vi "Comm String Send Command.vi"(0 "niDTS Comm String in":refnum<class "niDTS Comm String.lvclass">, 5 "Command":string, 7 "Args":string, 11 "error in (no error)":errorcluster) -> (4 "niDTS Comm String out":refnum<class "niDTS Comm String.lvclass">, 6 "Response":string, 15 "error out":errorcluster)   [LabVIEW 2015, in "niDTS CommLib.lvlib" / "niDTS Comm String.lvclass"]
uses:
  niDTS Comm String.lvclass
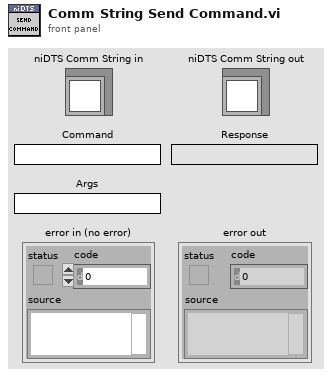
[diagram p1: front panel]
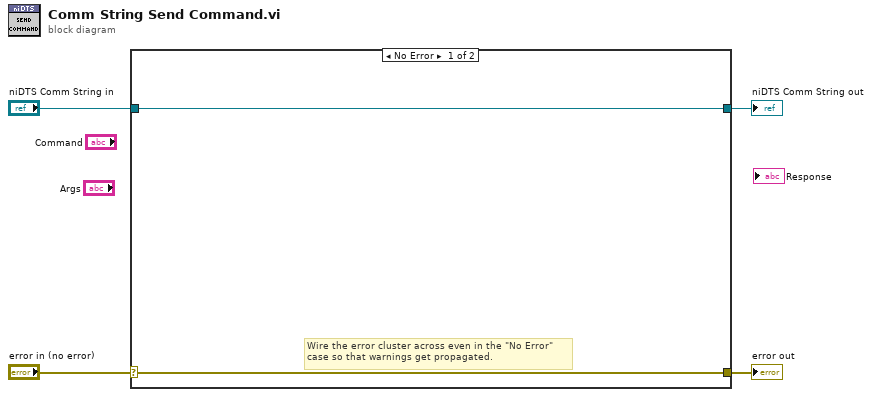
[diagram p0: block diagram]
diagram:
  n1 = case shown="No Error" "error in (no error)" {
    selector: "error in (no error)" -> [w5 w8]
    tunnel: [w5 w8] -> w3
    tunnel: [w6 w7] -> w1
    tunnel: "niDTS Comm String in" -> [w6 w7]
    frame No Error {
      # "Wire the error cluster across even in the \"No Error\"\ncase so that warnings get propagated."
    }
    frame Error {
    }
  }
  "error out" <- w3
  "niDTS Comm String out" <- w1
